vi "Write.vi"(8 "error in (no error)":errorcluster caption="错误输入（无错误）") -> (0 "error out":errorcluster caption="错误输出", 2 "布尔 3":bool)   [LabVIEW 2018]
panel:
  out "布尔 2":bool
  out "布尔":bool
  in  "确定":bool
  in  "取消":bool
  # "扫码完成后将模条放放夹具中，\n再按\"开始\"按键测试开始!!!"
  # "注意：按“取消后可重新扫条码”"
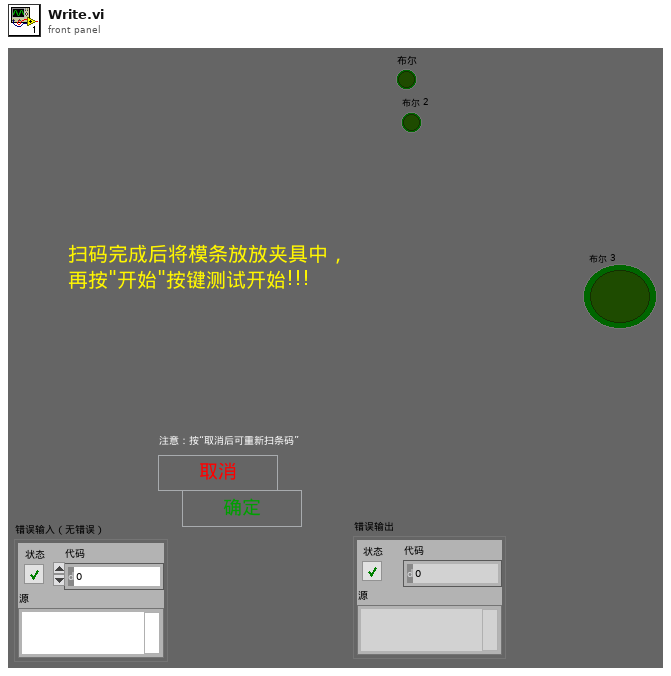
[diagram p1: front panel]
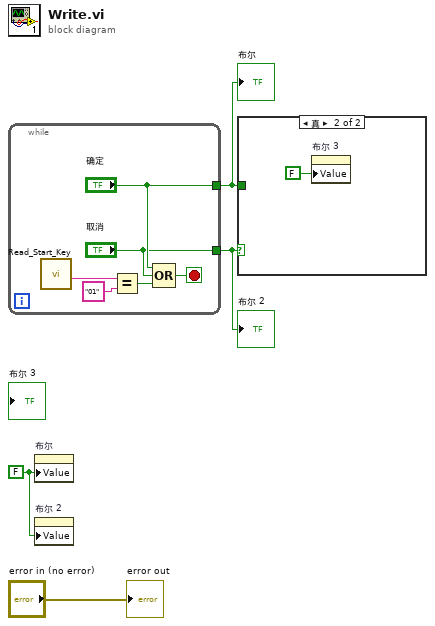
[diagram p0: block diagram]
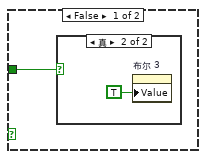
[diagram p2: hidden frame]
diagram:
  w3 = FALSE
  n1 = while {
    tunnel: ["确定"] -> w2
    tunnel: ["取消"] -> w1
    stop <- w7 stop-if-true
    n2 = call "Read_Start_Key.vi"() -> ("子字符串"=w10:string)  [unwired: 8 in, 3 out]
    n3 = Equal?(x=w10, y="01") -> (x = y?=w8:bool)
    n4 = Compound Arithmetic op=OR ("复合运算")("确定", "取消", w8) -> (w7:bool)
  }
  "布尔" <- w2
  "布尔 2" <- w1
  n5 = property on="布尔" class="Bool (严格)"("Value"=w3) -> ()  [unwired: 2 in, 2 out]
  n6 = property on="布尔 2" class="Bool (严格)"("Value"=w3) -> ()  [unwired: 2 in, 2 out]
  n7 = case shown="真" w1 {
    tunnel: w2 -> [w11 _]
    frame False {
      n8 = case shown="真" w11 {
        frame False {
        }
        frame True {
          n9 = property on="布尔 3" class="Bool (严格)"("Value"=TRUE ("布尔 3")) -> ()  [unwired: 2 in, 2 out]
        }
      }
    }
    frame True {
      n10 = property on="布尔 3" class="Bool (严格)"("Value"=FALSE ("布尔 3")) -> ()  [unwired: 2 in, 2 out]
    }
  }
  "error out" <- "error in (no error)"
